vi "UpdateOneStepIndex.vi"(8 "error in (no error)":errorcluster, 11 "StepIndexIn":u32) -> (0 "error out":errorcluster, 2 "OneStep?":bool, 3 "OneStepOut":u32)   [LabVIEW 2016, in "SeqProcessor.lvlib"]
uses:
  SeqProcessor.lvlib
  <vilib>/addons/PointValueMap/subVIs/Point_Write_variant.vi
  <vilib>/addons/PointValueMap/PointValueMap.lvlib
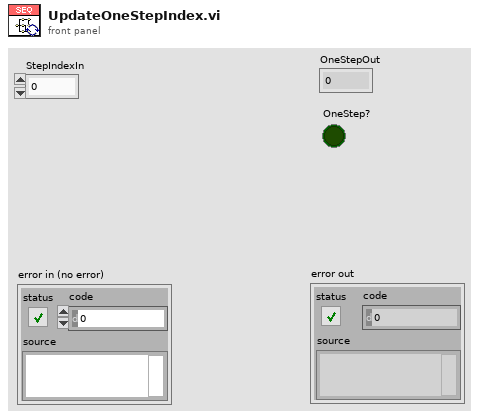
[diagram p1: front panel]
types:
  T1 = typedef "PointValueMap.lvlib/PointMap.ctl" = refnum<data-value>
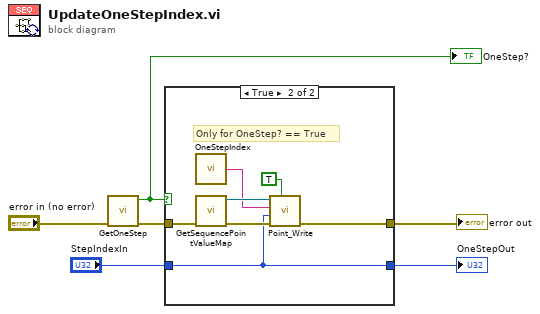
[diagram p0: block diagram]
diagram:
  n1 = call "GetOneStep.vi"("error in (no error)"="error in (no error)") -> ("error out"=w5:errorcluster, "OneStep?"=w2:bool)  [unwired: 8 in, 1 out]
  "OneStep?" <- w2
  n2 = case shown="True" w2 {
    tunnel: w5 -> [w8 w15]
    tunnel: [w8 w10] -> w4
    tunnel: "StepIndexIn" -> [w7 w9]
    tunnel: [w7 w9] -> w1
    frame False {
    }
    frame True {
      # "Only for OneStep? == True"
      n3 = call "OneStepIndex.vi"() -> ("OneStepIndex"=w12:string)  [unwired: 5 in]
      n4 = call "GetSequencePointValueMap.vi"("error in (no error)"=w15) -> ("error out"=w13:errorcluster, "SeqMap"=w14:T1)  [unwired: 9 in]
      n5 = call-poly <vilib>:"Point_Write.vi"("Auto Create?"=TRUE, "Error In"=w13, "Value"=w9, "Tag"=w12, "Map"=w14) -> ("Error Out"=w10:errorcluster)  [unwired: 5 in, 1 out]
    }
  }
  "error out" <- w4
  "OneStepOut" <- w1
